vi "From String.vi"(8 "error in (no error)":errorcluster, 9 "initial scan location":u32, 10 "String":string, 11 "Boolean in":refnum<class "Abs_Boolean.lvclass">) -> (0 "error out":errorcluster, 1 "offset past scan":u32, 2 "Remaining String":string, 3 "Boolean out":refnum<class "Abs_Boolean.lvclass">)   [LabVIEW 2021, in "Abs_Boolean.lvclass"]
uses:
  Abs_Boolean.lvclass
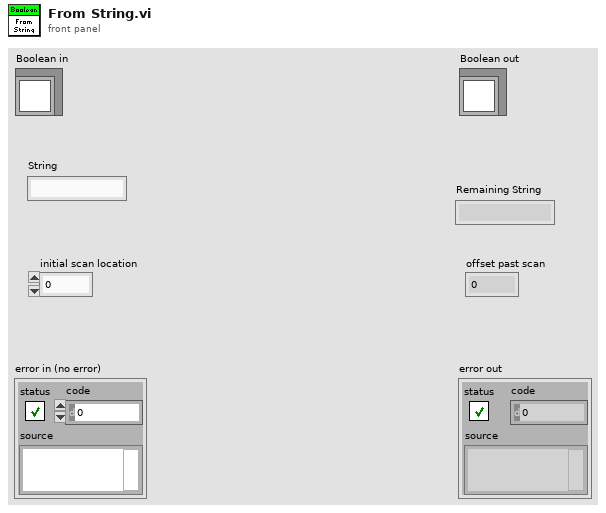
[diagram p1: front panel]
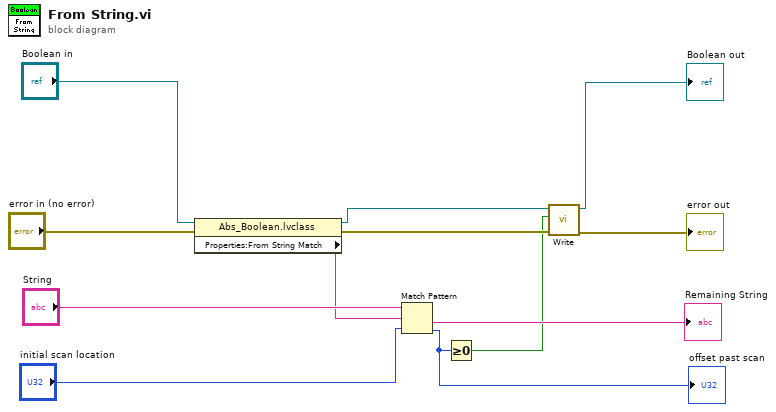
[diagram p0: block diagram]
diagram:
  n1 = property class="Abs_Boolean.lvclass"(reference="Boolean in", error in="error in (no error)") -> (reference out=w4:refnum<class "Abs_Boolean.lvclass">, error out=w5:errorcluster, "Properties:From String Match"=w3:string)
  n2 = Match Pattern(string="String", regular expression=w3, offset (0)="initial scan location") -> (after substring=→"Remaining String":string, offset past match=w2:i32)  [unwired: 2 out]
  "offset past scan" <- w2
  n3 = Greater Or Equal To 0?(x=w2) -> (x >= 0?=w1:bool)
  n4 = call-dynamic "Write.vi"("error in (no error)"=w5, "Boolean"=w1, "Boolean in"=w4) -> ("error out"=→"error out":errorcluster, "Boolean out"=→"Boolean out":refnum<class "Abs_Boolean.lvclass">)  [unwired: 7 in]
